vi "Write Multiple Digital Ports.vi"(8 "error in (no error)":errorcluster, 10 "Array":T1(array[cluster]), 11 "VISA resource name":refnum<visa-resource-name>) -> (0 "error out":errorcluster, 3 "VISA resource name out":refnum<visa-resource-name>)   [LabVIEW 2020, in "BDAQ-6104.lvlib"]
uses:
  <instrlib>/BDAQ-6104/BDAQ-6104.lvlib
panel:
  out "Command String":string
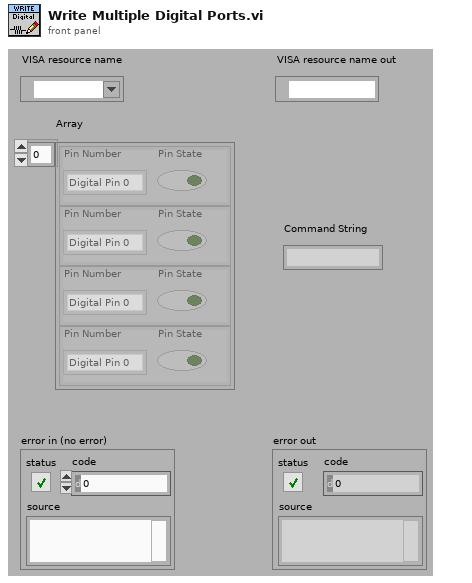
[diagram p1: front panel]
types:
  T1 = cluster{"Pin Number":enum16{"Digital Pin 0", "Digital Pin 1", "Digital Pin 2", "Digital Pin 3"}, "Pin State":bool}[]
  T2 = enum16{"Digital Pin 0", "Digital Pin 1", "Digital Pin 2", "Digital Pin 3"}
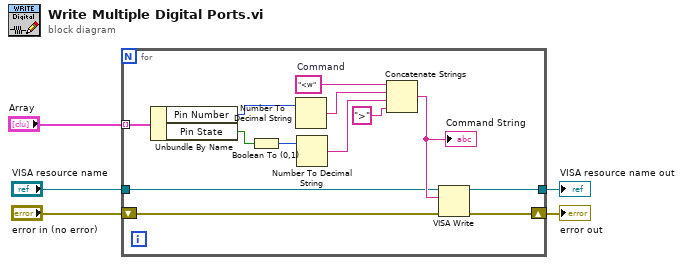
[diagram p0: block diagram]
diagram:
  n1 = for {
    tunnel: [w12] -> w5
    tunnel: "Array" -> [w9] mode=indexing
    tunnel: "VISA resource name" -> [w11]
    shift-right: [w6] -> w1
    shift-left: "error in (no error)" -> [w10]
    w17 = "<w"  # Command
    n2 = Unbundle By Name(w9) -> ("Pin Number"=w8:T2, "Pin State"=w7:bool)
    n3 = Boolean To (0,1)(Boolean=w7) -> (0, 1=w18:i16)
    n4 = Number To Decimal String(number=w8) -> (decimal integer string=w16:string)  [unwired: 1 in]
    n5 = Number To Decimal String(number=w18) -> (decimal integer string=w15:string)  [unwired: 1 in]
    n6 = Concatenate Strings(w17, w16, w15, ">" ("string")) -> (w13:string)
    "Command String" <- w13
    n7 = VISA Write(VISA resource name=w11, write buffer=w13, error in (no error)=w10) -> (VISA resource name out=w12:refnum<visa-resource-name>, error out=w6:errorcluster)  [unwired: 1 out]
  }
  "VISA resource name out" <- w5
  "error out" <- w1
